vi "SmartMotor_serial cmd-response.vi"(0 "VISA In":refnum<visa-resource-name>, 1 "mode":enum16{"wr & rd", "write", "read"}(ring), 3 "flush transcvr(F)":bool, 5 "cmd":string, 9 "ReadWait":u32=50, 11 "error in":errorcluster, 12 "Sem Timeout (5000)":i32=5000, 14 "MotorSpecifier(None)":T1) -> (4 "VISA out":refnum<visa-resource-name>, 6 "str out":string, 8 "cmd str out":string, 10 "timeout?":bool, 15 "error out":errorcluster)   [LabVIEW 2020]
doc: "Developed by: Kevin Thompson\nThompson Engineering\nkevin@thompsonengineering.net\n(510) 673-3614"
uses:
  TD SerialBusMotorSpecifier_enum.ctl
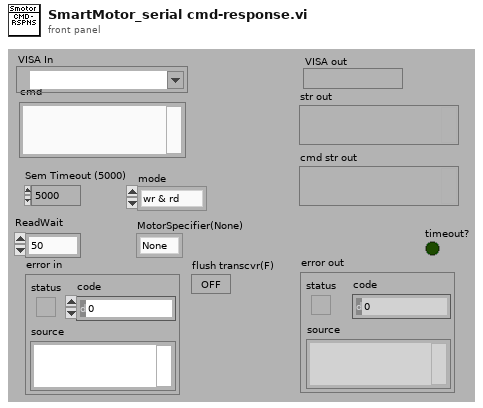
[diagram p1: front panel]
types:
  T1 = typedef "TD SerialBusMotorSpecifier_enum.ctl" = enum16{"None", "Global", "M1", "M2", "M3"}
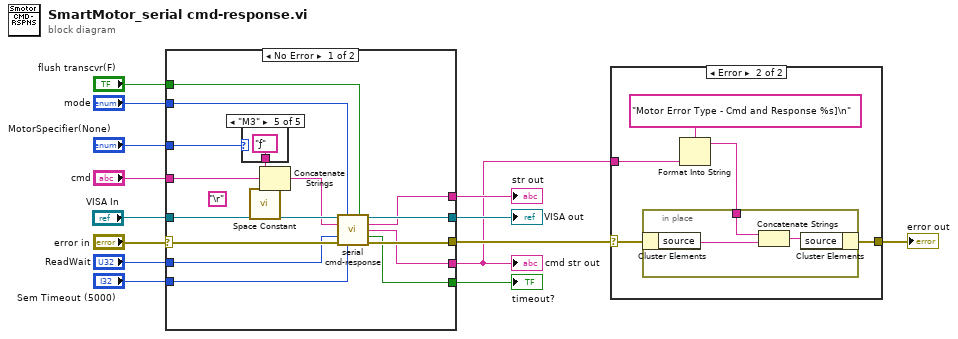
[diagram p0: block diagram]
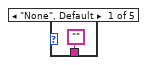
[diagram p3: hidden frame]
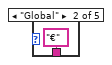
[diagram p4: hidden frame]
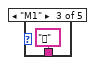
[diagram p5: hidden frame]
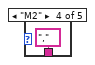
[diagram p6: hidden frame]
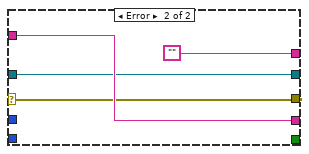
[diagram p7: hidden frame]
diagram:
  n1 = case shown="No Error" "error in" {
    selector: "error in" -> [w30 w38]
    tunnel: [w16 _] -> w4
    tunnel: [w18 ""] -> w5
    tunnel: [w19 w38] -> w3
    tunnel: "VISA In" -> [w29 w37]
    tunnel: "MotorSpecifier(None)" -> [w27 _]
    tunnel: "cmd" -> [w26 w39]
    tunnel: "mode" -> [w24 _]
    tunnel: "flush transcvr(F)" -> [w23 _]
    tunnel: "ReadWait" -> [w22 _]
    tunnel: "Sem Timeout (5000)" -> [w21 _]
    tunnel: [w20 w37] -> w6
    tunnel: [w17 w39] -> w1
    frame No Error {
      (unwired) "\r"
      n2 = case shown="\"M3\"" w27 {
        tunnel: ["" "€" "" "‚" "ƒ"] -> w28
        frame "None", Default {
        }
        frame "Global" {
        }
        frame "M1" {
        }
        frame "M2" {
        }
        frame "M3" {
        }
      }
      n3 = call <vilib>:"Space Constant.vi"() -> ("String"=w15:string)
      n4 = Concatenate Strings(w28, w26, w15) -> (w25:string)
      n5 = call "serial cmd-response.vi"("VISA In"=w29, "mode"=w24, "flush transcvr(F)"=w23, "cmd"=w25, "ReadWait"=w22, "error in"=w30, "Sem Timeout (5000)"=w21) -> ("VISA out"=w20:refnum<visa-resource-name>, "rsp str out"=w18:string, "cmd str out"=w17:string, "timeout?"=w16:bool, "error out"=w19:errorcluster)  [unwired: 4 in]
    }
    frame Error {
    }
  }
  "timeout?" <- w4
  "str out" <- w5
  "VISA out" <- w6
  "cmd str out" <- w1
  n6 = case shown="Error" w3 {
    selector: w3 -> [w40 w44]
    tunnel: [w40 w45] -> w2
    tunnel: w1 -> [_ w41]
    frame No Error {
    }
    frame Error {
      n7 = Format Into String(format string="Motor Error Type - Cmd and Response %s]\n", w41) -> (resulting string=w43:string)  [unwired: 2 in, 1 out]
      n8 = in-place {
        in-place-border: w43 -> [w47]
        n9 = in-place-cluster #1(w44) -> ("source"=w48:string)
        n10 = Concatenate Strings(w47, w48) -> (w46:string)
        n11 = in-place-cluster #1("source"=w46) -> (w45:errorcluster)
      }
    }
  }
  "error out" <- w2
